vi "Unbind.vi"(8 "error in":errorcluster, 10 "endpoint":string, 11 "socket in":refnum<class "Socket.lvclass">) -> (0 "error out":errorcluster, 3 "socket out":refnum<class "Socket.lvclass">)   [LabVIEW 2025, in "ZeroMQ.lvlib" / "Socket.lvclass"]
doc: "Unbinds a socket from a particular <b>endpoint</b>. Opposite of zmq_bind. Use zmq_close to unbind from all endpoints.\n\nDetailed API documentation: http://api.zeromq.org/3-2:zmq-unbind"
uses:
  Socket.lvclass
  Socket.lvclass/Socket.ctl
  <vilib>/Utility/error.llb/Error Cluster From Error Code.vi
  libzmq-v143-mt-4_3_6/LibZMQ.lvlib
panel:
  # "ØMQ"
  # "labview"
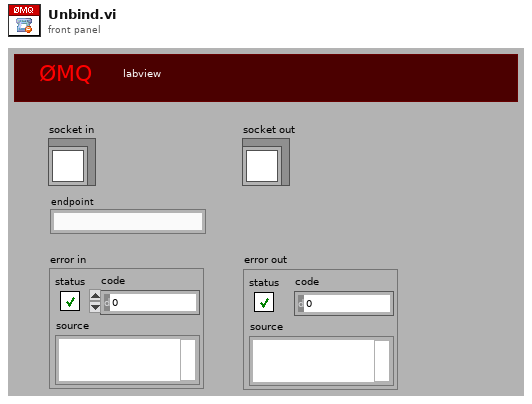
[diagram p1: front panel]
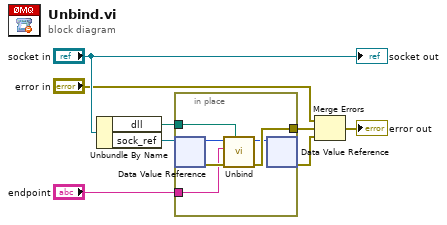
[diagram p0: block diagram]
diagram:
  n1 = Unbundle By Name("socket in") -> ("dll"=w1:path, "sock_ref"=w5:refnum<data-value>)
  n2 = in-place {
    in-place-border: "endpoint" -> [w12]
    in-place-border: [w13] -> w7
    in-place-border: w1 -> [w9]
    n3 = in-place-dvr #1(w5) -> (w11:u64, w14:errorcluster)
    n4 = call "Unbind.vi"("path override"=w9, "error in (no error)"=w14, "addr_"=w12, "s_"=w11) -> ("error out"=w13:errorcluster, "s_ out"=w10:u64)  [unwired: 6 in]
    n5 = in-place-dvr #1(w10) -> (w2:errorcluster)  [unwired: 1 out]
  }
  n6 = Merge Errors("error in", w7, w2) -> (→"error out":errorcluster)
  "socket out" <- "socket in"
